vi "List Linked List Roots.vi"(8 "error in (no error)":errorcluster, 11 "Linked List Ref":refnum<data-value>) -> (0 "error out":errorcluster, 1 "Root Names":string[](array[string]), 2 "Root IDs":string[](array[string]), 3 "Linked List Ref out":refnum<data-value>)   [LabVIEW 2020, in "Linked Lists.lvlib" / "Linked List Ref.lvclass"]
uses:
  <vilib>/gpm_packages/@cs/linked-list/Source/Linked List/Linked List Ref/Linked List Ref.lvclass
  <vilib>/gpm_packages/@cs/linked-list/Source/Linked List/ILinkedList/ILinked List.lvclass
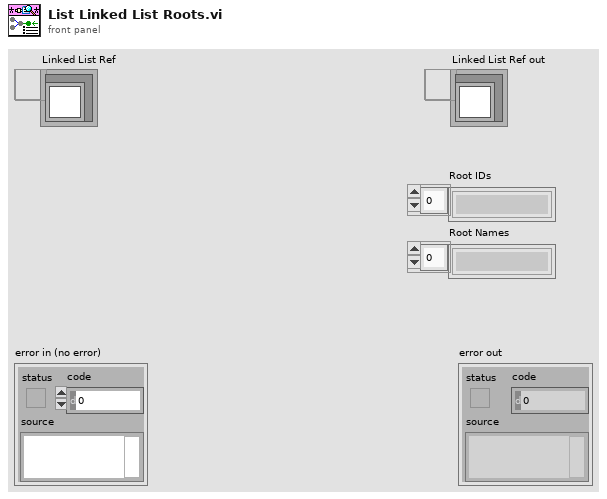
[diagram p1: front panel]
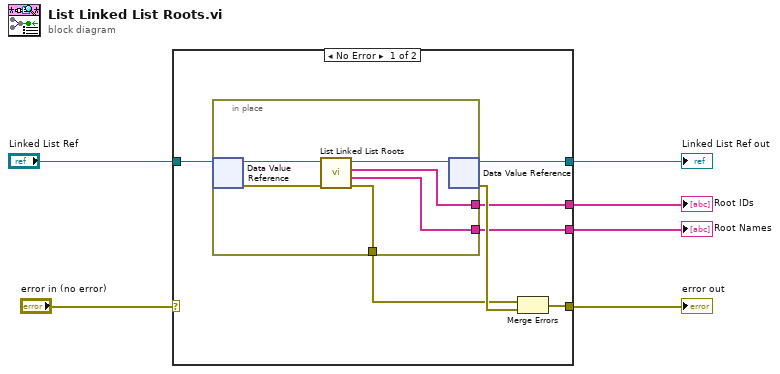
[diagram p0: block diagram]
diagram:
  n1 = case shown="No Error" "error in (no error)" {
    selector: "error in (no error)" -> [_ w20]
    tunnel: "Linked List Ref" -> [w13 w21]
    tunnel: [w12 w21] -> w5
    tunnel: [w11 w20] -> w3
    tunnel: [w8 _] -> w2
    tunnel: [w7 _] -> w1
    frame No Error {
      n2 = in-place {
        in-place-border: [w16] -> w9
        in-place-border: [w15] -> w8
        in-place-border: [w14] -> w7
        n3 = in-place-dvr #1(w13) -> (w19:refnum<class "ILinked List.lvclass">, w17:errorcluster)
        n4 = call-dynamic "List Linked List Roots.vi"("error in (no error)"=w17, "ILinked List in"=w19) -> ("error out"=w16:errorcluster, "Root Names"=w14:string[], "Root IDs"=w15:string[], "ILinked List out"=w18:refnum<class "ILinked List.lvclass">)  [unwired: 6 in]
        n5 = in-place-dvr #1(w18) -> (w12:refnum<data-value>, w10:errorcluster)
      }
      n6 = Merge Errors(w9, w10) -> (w11:errorcluster)
    }
    frame Error {
    }
  }
  "error out" <- w3
  "Linked List Ref out" <- w5
  "Root IDs" <- w2
  "Root Names" <- w1
